vi "DashboardGetPolyscopeVersion.vi"(8 "Dashboard":refnum<k24>, 11 "error in":errorcluster) -> (0 "Response":cluster{"Message":string, "Succeed":bool}, 1 "Version":T1, 3 "error out":errorcluster)   [LabVIEW 2022 SP3, in "UnderAutomation.UniversalRobots.lvlib"]
uses:
  UnderAutomation.UniversalRobots.lvlib
  C:/Users/fg/Documents/UniversalRobots.vi/LabVIEW_2023/UnderAutomation.UniversalRobots/lib/UnderAutomation.UniversalRobots.dll
  LabVIEW_2023/UnderAutomation.UniversalRobots/lib/UnderAutomation.UniversalRobots.dll
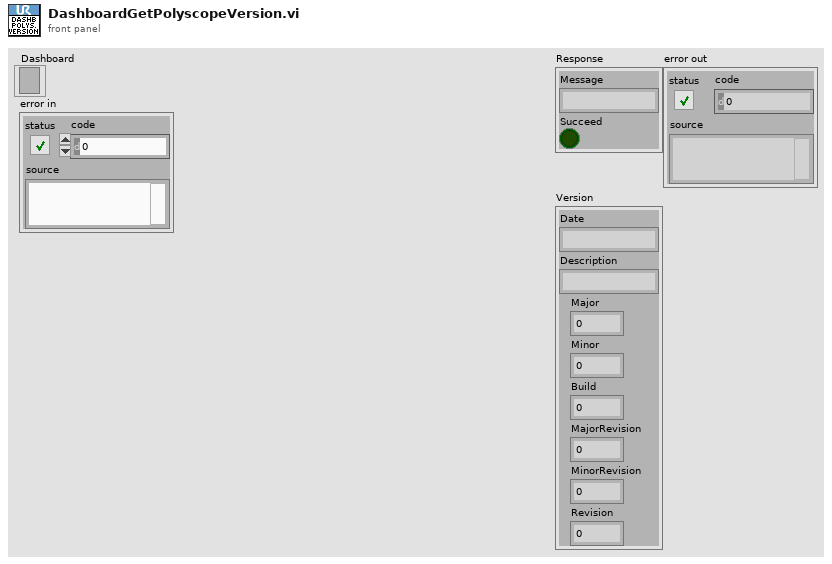
[diagram p1: front panel]
types:
  T1 = cluster{"Date":string, "Description":string, "Major":i32, "Minor":i32, "Build":i32, "MajorRevision":i16, "MinorRevision":i16, "Revision":i32}
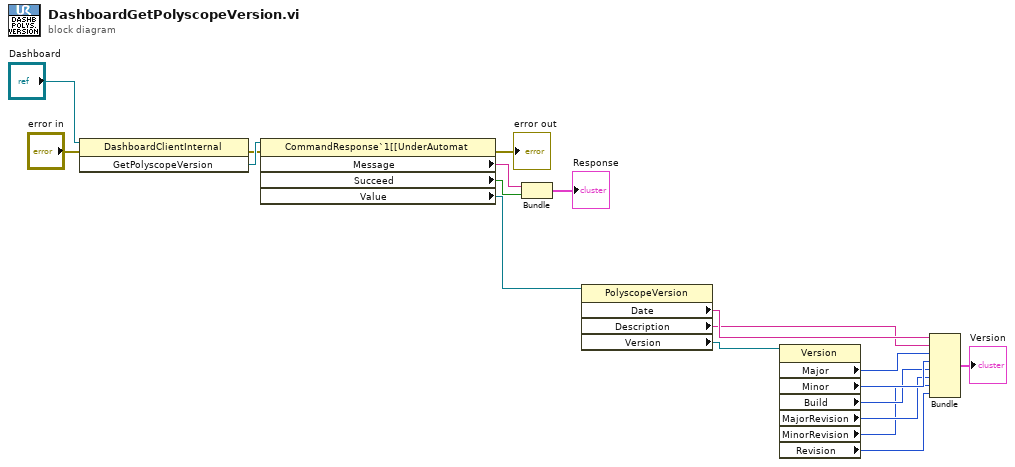
[diagram p0: block diagram]
diagram:
  n1 = invoke class="DashboardClientInternal" method="GetPolyscopeVersion"(reference="Dashboard", error in="error in") -> (error out=w13:errorcluster, "GetPolyscopeVersion"=w18:refnum<k24>)  [unwired: 1 in, 1 out]
  n2 = property class="CommandResponse`1[[UnderAutomat"(reference=w18, error in=w13) -> (error out=→"error out":errorcluster, "Message"=w17:string, "Succeed"=w16:bool, "Value"=w11:refnum<k24>)  [unwired: 1 out]
  n3 = Bundle("Message"=w17, "Succeed"=w16) -> (→"Response":cluster{"Message":string, "Succeed":bool})  [unwired: 1 in]
  n4 = property class="PolyscopeVersion"(reference=w11) -> ("Date"=w9:string, "Description"=w8:string, "Version"=w10:refnum<k24>)  [unwired: 1 in, 2 out]
  n5 = property class="Version"(reference=w10) -> ("Major"=w7:i32, "Minor"=w6:i32, "Build"=w5:i32, "MajorRevision"=w4:i16, "MinorRevision"=w3:i16, "Revision"=w2:i32)  [unwired: 1 in, 2 out]
  n6 = Bundle("Date"=w9, "Description"=w8, "Major"=w7, "Minor"=w6, "Build"=w5, "MajorRevision"=w4, "MinorRevision"=w3, "Revision"=w2) -> (→"Version":T1)  [unwired: 1 in]
